vi "Write Point.vi"(3 "(FPPos)":refnum<class "Point_FPPos.lvclass">, 4 "Point":T1) -> (5 "(FPPos) Out":refnum<class "Point_FPPos.lvclass">)   [LabVIEW 2020, in "Point_FPPos.lvclass"]
uses:
  Point_FPPos.lvclass
  TypeDefs_Utility/Cluster_Pos_Top Left position.ctl
  Point_FPPos.lvclass/Point_FPPos.ctl
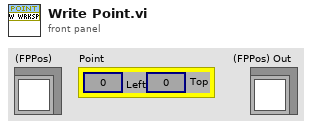
[diagram p1: front panel]
types:
  T1 = typedef "Cluster_Pos_Top Left position.ctl" = cluster{"Left":i16, "Top":i16}
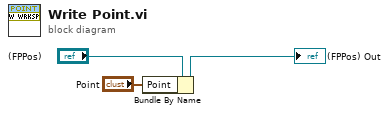
[diagram p0: block diagram]
diagram:
  n1 = Bundle By Name(cluster="(FPPos)", "Point"="Point") -> (→"(FPPos) Out":refnum<class "Point_FPPos.lvclass">)
